vi "Get 1D Array Double Complex.vi"(5 "use temporary file? (F)":bool, 7 "data type of variable":cdb[](array[numeric]), 8 "error in":errorcluster, 10 "variable name":string, 11 "GOLPI ref. in":T1={"pipe handle"={"lv_proc.dll file path"=path "", "process instance handle"=[], "debug mode"=FALSE, "debug data"=[]}, "fast read timeout [ms]"=500, "fast read settle time [ms]"=10, "fast read to multiple [ms]"=1, "max elements per input line"=100, "slow read timeout [ms]"=5000, "stdin double format specifier"="%_16e", "max elements per stdout output column"=100, "console mode bitstream"=FALSE, "bitstream first read timeout [ms]"=1000, "bitstream read timeout [ms]"=50, "struct transfer possible"=FALSE, "matlab mode"=FALSE}) -> (0 "error out":errorcluster, 2 "value":cdb[](array[numeric]) format="%.2f", 3 "GOLPI ref. out":T1={"pipe handle"={"lv_proc.dll file path"=path "", "process instance handle"=[], "debug mode"=FALSE, "debug data"=[]}, "fast read timeout [ms]"=500, "fast read settle time [ms]"=10, "fast read to multiple [ms]"=1, "max elements per input line"=100, "slow read timeout [ms]"=5000, "stdin double format specifier"="%_16e", "max elements per stdout output column"=100, "console mode bitstream"=FALSE, "bitstream first read timeout [ms]"=1000, "bitstream read timeout [ms]"=50, "struct transfer possible"=FALSE, "matlab mode"=FALSE})   [LabVIEW 2020, in "GOLPI library.lvlib"]
doc: "Part of polymorph Get Variable.vi"
uses:
  GOLPI library.lvlib
  GOLPI reference Type Def.ctl
  Pipe Handle.ctl
  Bitstream Data Type.ctl
  Custom Error Codes Enum Type Def.vi
  LV Process library.lvlib
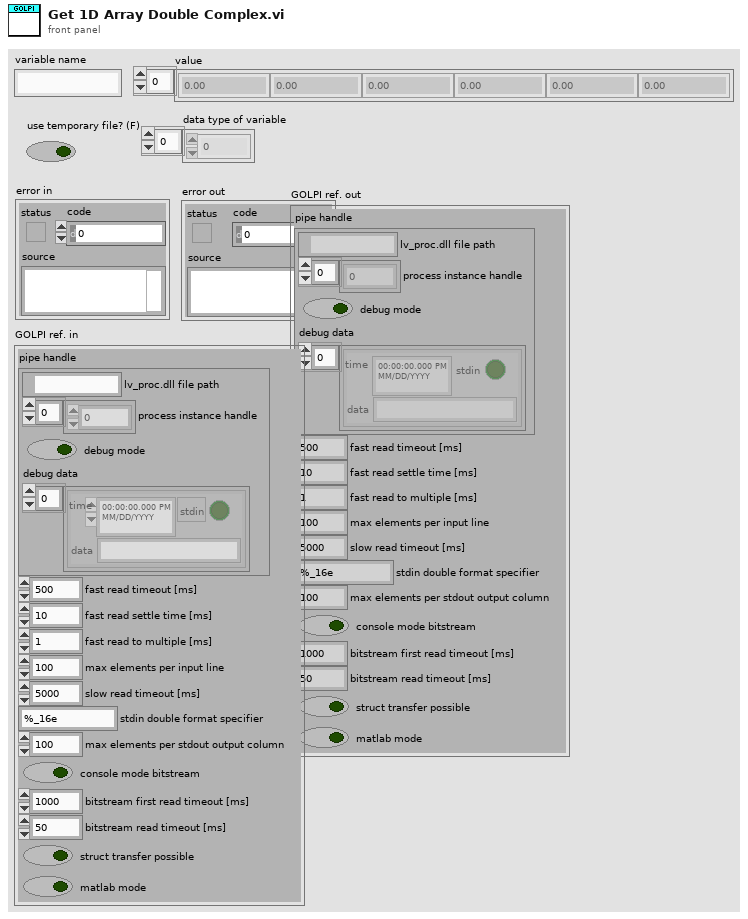
[diagram p1: front panel]
types:
  T1 = typedef "GOLPI library.lvlib/GOLPI reference Type Def.ctl" = cluster{"pipe handle":T2, "fast read timeout [ms]":u32, "fast read settle time [ms]":u32, "fast read to multiple [ms]":u32, "max elements per input line":u32, "slow read timeout [ms]":u32, "stdin double format specifier":string, "max elements per stdout output column":u32, "console mode bitstream":bool, "bitstream first read timeout [ms]":u32, "bitstream read timeout [ms]":u32, "struct transfer possible":bool, "matlab mode":bool}
  T2 = typedef "LV Process library.lvlib/Pipe Handle.ctl" = cluster{"lv_proc.dll file path":path, "process instance handle":u32[], "debug mode":bool, "debug data":cluster{"time":timestamp, "stdin":bool, "data":string}[]}
  T3 = typedef "GOLPI library.lvlib/Bitstream Data Type.ctl" = enum16{"dummy", "int", "uint", "float", "complex", "str", "real numeric"}
  T4 = typedef "GOLPI library.lvlib/Custom Error Codes Enum Type Def.vi" = enum16{"no error", "00 working directory PAR1 missing", "01 octave binary PAR1 missing", "02 octave report error PAR1", "03 empty output last cmd PAR1", "04 missing temporary file PAR1", "05 pwd PAR 1 not exist", "06 oct package not installed", "07 octave default binary missing", "10 var PAR1 not string, vect", "11 var PAR1 not num, scal, ~compl", "12 var PAR1 not num, scal, compl", "13 var PAR1 not num, vect, ~compl", "14 var PAR1 not num, vect, compl", "15 var PAR1 not num, mat, ~compl", "16 var PAR1 not num, mat, ~compl", "30 read timeout", "60 bitstream transport failed", "61 bitstream decode error PAR1", "62 bitstream cannot be set", "70 struct transfer not possible", "80 struct: cluster elem. PAR1 not implem.", "81 struct: structure field PAR1 not implem.", "82 struct: size mismatch of PAR1", "83 struct: type mismatch of PAR1", "98 internal error", "99 not finished", "90 Not supported in Matlab mode", "91 Matlab variable transfer error", "92 Matlab Script Error"}
  T5 = typedef "GOLPI library.lvlib/Bitstream Data.ctl" = cluster{"double":dbl[][], "cplx double":cdb[][], "int64":i64[][], "uint64":u64[][], "str":string[], "data type":T3}
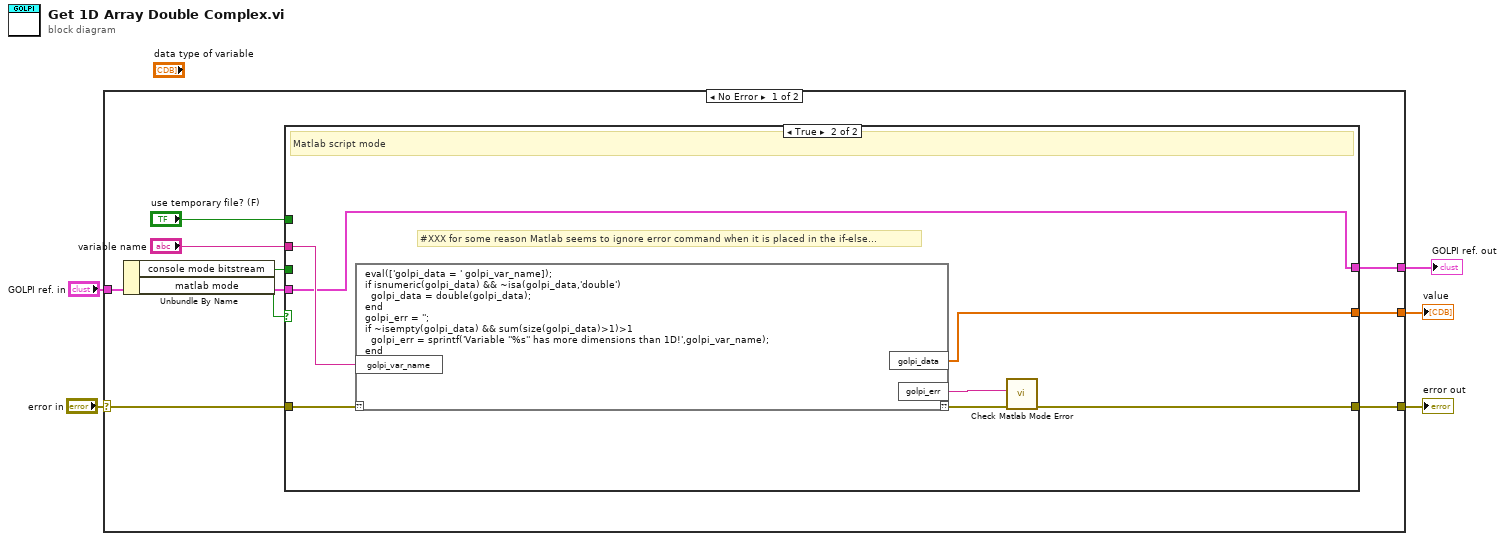
[diagram p0: block diagram]
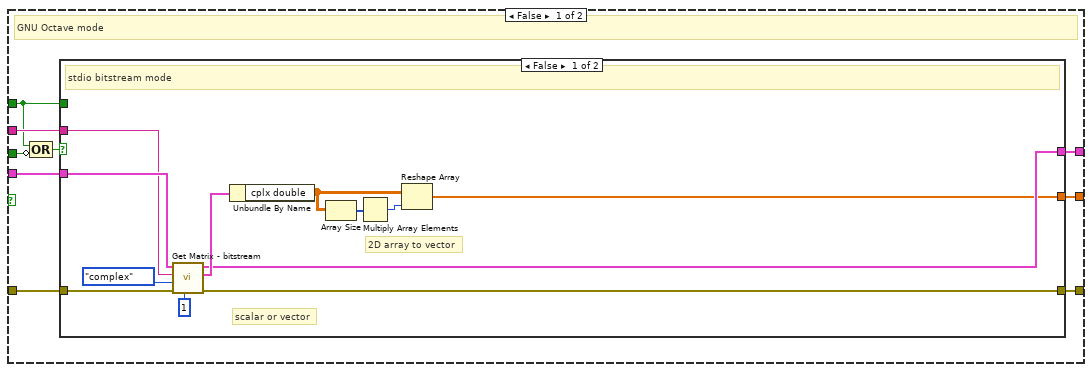
[diagram p2: hidden frame]
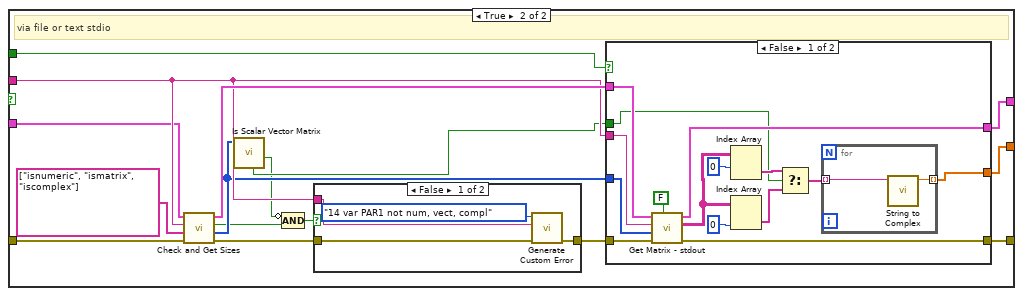
[diagram p3: hidden frame]
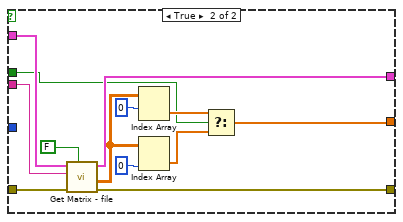
[diagram p4: hidden frame]
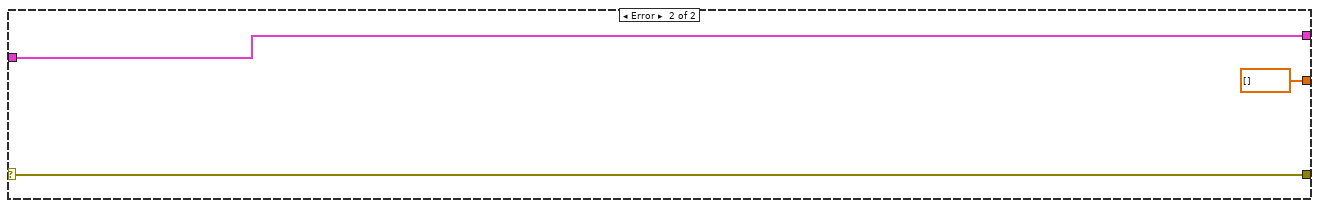
[diagram p6: hidden frame]
diagram:
  n1 = case shown="No Error" "error in" {
    selector: "error in" -> [w14 w96]
    tunnel: [w13 w96] -> w5
    tunnel: [w11 cdb[] [] ("value")] -> w3
    tunnel: "GOLPI ref. in" -> [w9 w94]
    tunnel: [w10 w94] -> w1
    frame No Error {
      n2 = Unbundle By Name(w9) -> ("console mode bitstream"=w8:bool, "matlab mode"=w6:bool)
      n3 = case shown="True" w6 {
        tunnel: w14 -> [w23 w93]
        tunnel: [w22 w87] -> w13
        tunnel: "variable name" -> [w21 w92]
        tunnel: [w20 w90] -> w11
        tunnel: [w19 w91] -> w10
        tunnel: w9 -> [w18 w91]
        tunnel: w8 -> [w17 _]
        tunnel: "use temporary file? (F)" -> [w16 _]
        frame False {
          # "GNU Octave mode"
          n4 = Compound Arithmetic op=OR(w16, invert w17) -> (w15:bool)
          n5 = case shown="False" w15 {
            tunnel: w23 -> [w35 w51]
            tunnel: [w30 w46] -> w22
            tunnel: w21 -> [w33 w45]
            tunnel: [w24 w44] -> w20
            tunnel: w16 -> [_ w43]
            tunnel: w18 -> [w34 w40]
            tunnel: [w25 w39] -> w19
            frame False {
              # "scalar or vector"
              # "2D array to vector"
              # "stdio bitstream mode"
              n6 = call "Get Matrix - bitstream.vi"("max dimensions (0: scalar)"=1, "error in (no error)"=w35, "data type"=Bitstream_Data_Type."complex", "variable name"=w33, "GOLPI ref. in"=w34) -> ("error out"=w30:errorcluster, "data"=w26:T5, "GOLPI ref. out"=w25:T1)  [unwired: 4 in]
              n7 = Unbundle By Name(w26) -> ("cplx double"=w29:cdb[][])
              n8 = Array Size(array=w29) -> (size(s)=w28:i32[])
              n9 = Multiply Array Elements(1:w28) -> (0:w27:i32)
              n10 = Reshape Array(w29, w27) -> (w24:cdb[])
            }
            frame True {
              # "via file or text stdio"
              n11 = call "Check and Get Sizes.vi"("error in (no error)"=w51, "test commands"=string[] ["isnumeric", "ismatrix", "iscomplex"], "variable name"=w45, "GOLPI ref. in"=w40) -> ("error out"=w50:errorcluster, "octave sizes"=w42:i32[], "all tests OK?"=w38:bool, "GOLPI ref. out"=w48:T1)  [unwired: 4 in]
              n12 = call "Is Scalar Vector Matrix.vi"("octave sizes"=w42) -> ("is matrix?"=w36:bool, "row vector?"=w41:bool)  [unwired: 5 in, 4 out]
              n13 = Compound Arithmetic op=AND(invert w36, w38) -> (w37:bool)
              n14 = case shown="False" w37 {
                tunnel: w50 -> [w84 w86]
                tunnel: [w83 w86] -> w47
                tunnel: w45 -> [w82 _]
                frame False {
                  n15 = call "Generate Custom Error.vi"("error in"=w84, "PAR1"=w82, "GOLPI error"=Custom_Error_Codes_Enum_Type_Def.vi."14 var PAR1 not num, vect, compl" ("Enum")) -> ("error out"=w83:errorcluster)  [unwired: 8 in]
                }
                frame True {
                }
              }
              n16 = case shown="False" w43 {
                tunnel: w48 -> [w66 w73]
                tunnel: [w65 w74] -> w39
                tunnel: w47 -> [w63 w76]
                tunnel: [w64 w75] -> w46
                tunnel: w42 -> [w62 _]
                tunnel: w41 -> [w52 w69]
                tunnel: w45 -> [w61 w70]
                tunnel: [w59 w71] -> w44
                frame False {
                  n17 = call "Get Matrix - stdout.vi"("is string?"=FALSE ("is string"), "error in (no error)"=w63, "octave sizes"=w62, "variable name"=w61, "GOLPI ref. in"=w66) -> ("error out"=w64:errorcluster, "array"=w53:string[][], "GOLPI ref. out"=w65:T1)  [unwired: 4 in]
                  n18 = Index Array(array=w53, index (row)=0) -> (element=w56:string[])  [unwired: 1 in]
                  n19 = Index Array(array=w53, index (col)=0 ("disabled index (col)")) -> (element=w55:string[])  [unwired: 1 in]
                  n20 = Select(t=w56, s=w52, f=w55) -> (s? t:f=w54:string[])
                  n21 = for {
                    tunnel: w54 -> [w68] mode=indexing
                    tunnel: [w67] -> w59 mode=indexing
                    n22 = call "String to Complex.vi"("string"=w68) -> ("complex number"=w67:cdb)  [unwired: 10 in]
                  }
                }
                frame True {
                  n23 = call "Get Matrix - file.vi"("is string?"=FALSE ("is string"), "error in (no error)"=w76, "variable name"=w70, "GOLPI ref. in"=w73) -> ("error out"=w75:errorcluster, "cmplx double array"=w72:cdb[][], "GOLPI ref. out"=w74:T1)  [unwired: 3 in, 2 out]
                  n24 = Index Array(array=w72, index (row)=0) -> (element=w79:cdb[])  [unwired: 1 in]
                  n25 = Index Array(array=w72, index (col)=0 ("disabled index (col)")) -> (element=w78:cdb[])  [unwired: 1 in]
                  n26 = Select(t=w79, s=w69, f=w78) -> (s? t:f=w71:cdb[])
                }
              }
            }
          }
        }
        frame True {
          # "#XXX for some reason Matlab seems to ignore error command when it is placed in the if-else..."
          # "Matlab script mode"
          n27 = script code="eval(['golpi_data = ' golpi_var_name]);\nif isnumeric(golpi_data) && ~isa(golpi_data,'double')\n  golpi_data = double(golpi_data);\nend\ngolpi_err = '';\nif ~isempty(golpi_data) && sum(size(golpi_data)>1)>1\n  golpi_err = sprintf('Variable ''%s'' has more dimensions than 1D!',golpi_var_name);\nend"("??"=w93, "golpi_var_name"=w92) -> ("??"=w89:errorcluster, "golpi_data"=w90:cdb[], "golpi_err"=w88:string)
          n28 = call "Check Matlab Mode Error.vi"("error in"=w89, "custom error string (empty)"=w88) -> ("error out"=w87:errorcluster)  [unwired: 9 in]
        }
      }
    }
    frame Error {
    }
  }
  "value" <- w3
  "error out" <- w5
  "GOLPI ref. out" <- w1
